vi "Test Intensity Graph to ITX Graph.vi"() -> ()   [LabVIEW 2019]
uses:
  LV-Data.ITX/LV-Data.ITX.lvclass
panel:
  out "Intensity Graph":dbl[][](graph)
  out "file":path=path "C:/Users/voodoo.SEAGATE/Desktop/datatest/datatest.000019.itx"
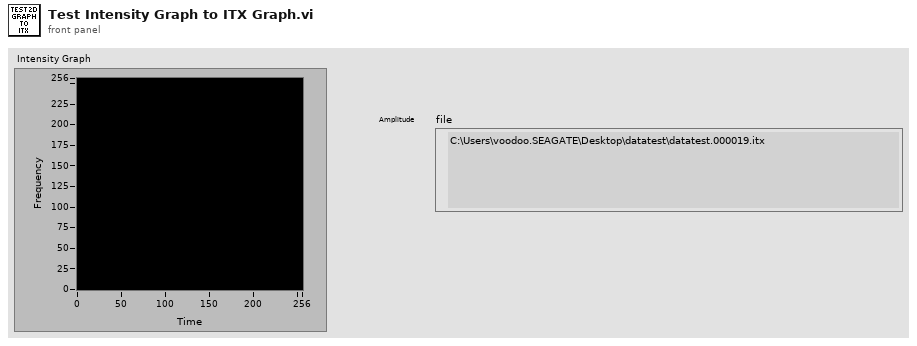
[diagram p1: front panel]
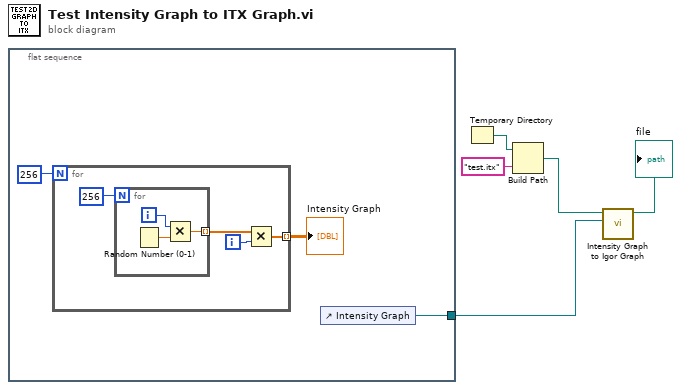
[diagram p0: block diagram]
diagram:
  n1 = flat-sequence {
    tunnel: [w6] -> w1
    frame #0 {
      n2 = for {
        N: 256 -> [_]
        tunnel: [w9] -> w7 mode=indexing
        i -> [w11]
        n3 = for {
          N: 256 -> [_]
          tunnel: [w13] -> w10 mode=indexing
          i -> [w15]
          n4 = Random Number (0-1)() -> (number: 0 to 1=w14:dbl)
          n5 = Multiply(x=w15, y=w14) -> (x*y=w13:dbl)
        }
        n6 = Multiply(x=w10, y=w11) -> (x*y=w9:dbl[])
      }
      "Intensity Graph" <- w7
      n7 = control-ref of="Intensity Graph"() -> (w6:refnum<vi>)
    }
  }
  n8 = Temporary Directory() -> (w4:path)
  n9 = Build Path(base path=w4, name or relative path="test.itx") -> (appended path=w3:path)
  n10 = call "Intensity Graph to Igor Graph.vi"("Intensity Graph Reference"=w1, "Path"=w3) -> ("file"=→"file":path)  [unwired: 8 in, 1 out]
